vi "coriolistest.vi"() -> ()   [LabVIEW 2021]
uses:
  CoriFlowBFS1Plus_class/CoriFlowBFS1Plus.lvclass
panel:
  in  "Filter(0-1)Min-Max":dbl=1.0 format="%#_13g"
  out "Temperature(C)":sgl
  out "FLow(ul/min)":sgl
  out "Density_g_L":sgl
  in  "VISA resource name":refnum<visa-resource-name>
  in  "stop":bool
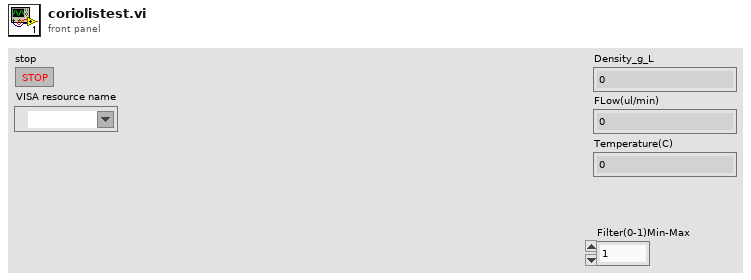
[diagram p1: front panel]
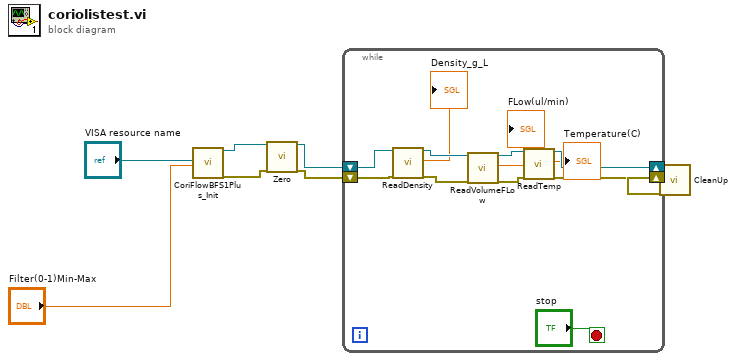
[diagram p0: block diagram]
diagram:
  n1 = call "CoriFlowBFS1Plus_Init.vi"("VISA resource name"="VISA resource name", "Filter(0-1)Min-Max"="Filter(0-1)Min-Max") -> ("object out"=w8:refnum<class "CoriFlowBFS1Plus.lvclass">, "error out"=w5:errorcluster)  [unwired: 16 in]
  n2 = call-dynamic "Zero.vi"("object in"=w8, "error in (no error)"=w5) -> ("object out"=w7:refnum<class "CoriFlowBFS1Plus.lvclass">, "error out"=w4:errorcluster)  [unwired: 16 in]
  n3 = while {
    shift-right: [w17] -> w6
    shift-left: w7 -> [w20]
    shift-right: [w13] -> w3
    shift-left: w4 -> [w16]
    stop <- "stop" stop-if-true
    n4 = call-dynamic "ReadDensity.vi"("object in"=w20, "error in (no error)"=w16) -> ("object out"=w19:refnum<class "CoriFlowBFS1Plus.lvclass">, "Density_g_L"=→"Density_g_L":sgl, "error out"=w15:errorcluster)  [unwired: 15 in]
    n5 = call-dynamic "ReadVolumeFLow.vi"("object in"=w19, "error in (no error)"=w15) -> ("object out"=w18:refnum<class "CoriFlowBFS1Plus.lvclass">, "FLow(ul/min)"=→"FLow(ul/min)":sgl, "error out"=w14:errorcluster)  [unwired: 15 in]
    n6 = call-dynamic "ReadTemp.vi"("object in"=w18, "error in (no error)"=w14) -> ("object out"=w17:refnum<class "CoriFlowBFS1Plus.lvclass">, "Temperature(C)"=→"Temperature(C)":sgl, "error out"=w13:errorcluster)  [unwired: 15 in]
  }
  n7 = call-dynamic "CleanUp.vi"("object in"=w6, "error in (no error)"=w3) -> ()  [unwired: 16 in, 2 out]
